vi "openLoopControlView.vi"(10 "UserEvents in":refnum<class "UserEvents.lvclass">) -> ()   [LabVIEW 2015, in "FAMTViews.lvlib"]
uses:
  FAMTViews.lvlib
  UserEvents/UserEvents.lvclass
  CommandFactory/CommandFactory.lvclass
  UserEvents/UserEvents.lvclass/UserEvents.ctl
  Typedefs/StateSelector.ctl
  Commands/StartOpenLoopScan/StartOpenLoopScan.lvclass
  Typedefs/CommandSelector.ctl
  Typedefs/FAMTTypedefs.lvlib
panel:
  in  "cancelOpenLoopScanIsTrue":bool
  in  "startOpenLoopScanIsTrue":bool
  in  "Center Point":dbl[unit]
  in  "Force Setpoint":dbl[unit]
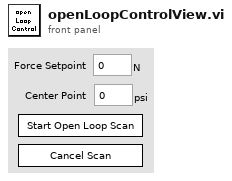
[diagram p1: front panel]
types:
  T1 = typedef "FAMTTypedefs.lvlib/PubDataEvents.ctl" = cluster{"State":refnum<user-event>, "ErrorCode":refnum<user-event>, "OutputData":refnum<user-event>, "InputData":refnum<user-event>, "ControllerData":refnum<user-event>, "TestStatus":refnum<user-event>, "LogPath":refnum<user-event>}
  T2 = typedef "FAMTTypedefs.lvlib/SubDataEvents.ctl" = cluster{"Command":refnum<user-event>}
  T3 = cluster{"Event Registration Refnum":refnum<event-registration>}
  T4 = typedef "FAMTTypedefs.lvlib/StateSelector.ctl" = enum16{"OfflineState", "FaultState", "StandbyState", "DisabledState", "EnabledState", "WaitForUserInputState", "PerformOpenLoopScanState"}
  T5 = typedef "FAMTTypedefs.lvlib/CommandSelector.ctl" = enum16{"Start", "Enable", "Disable", "Standby", "Shutdown"}
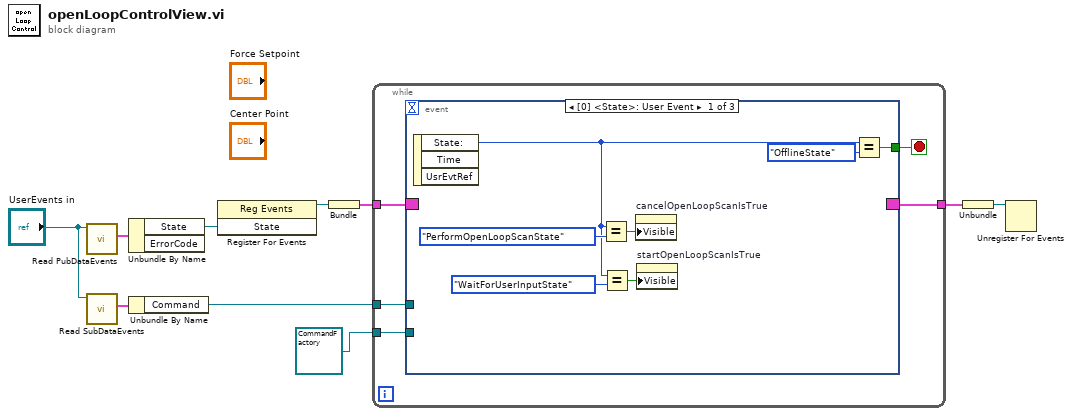
[diagram p0: block diagram]
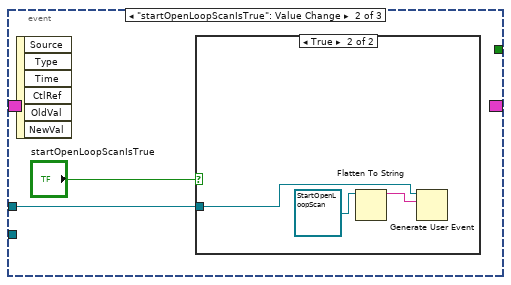
[diagram p2: hidden frame]
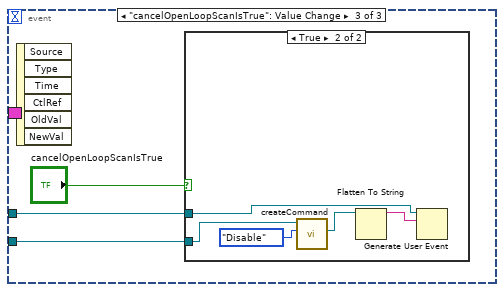
[diagram p4: hidden frame]
diagram:
  n1 = call "Read PubDataEvents.vi"("UserEvents in"="UserEvents in") -> ("PubDataEvents"=w10:T1)  [unwired: 9 in, 1 out]
  n2 = call "Read SubDataEvents.vi"("UserEvents in"="UserEvents in") -> ("SubDataEvents"=w4:T2)  [unwired: 9 in, 1 out]
  n3 = Unbundle By Name(w10) -> ("State"=w9:refnum<user-event>)  [unwired: 1 out]
  n4 = Unbundle By Name(w4) -> ("Command"=w2:refnum<user-event>)
  n5 = register-events(w9) -> (reference out=w8:refnum<event-registration>)  [unwired: 2 in, 1 out]
  n6 = Bundle("Event Registration Refnum"=w8) -> (w5:T3)  [unwired: 1 in]
  n7 = while {
    tunnel: w5 -> [w15]
    tunnel: [w14] -> w6
    tunnel: w2 -> [w12]
    tunnel: refnum<class "CommandFactory.lvclass"> refnum ("CommandFactory.lvclass") -> [w11]
    stop <- w13 stop-if-true
    n8 = event shown="[0] <State>: User Event" {
      selector: w15 -> [_ _ _]
      dyn-events: [_ _ _] -> w14
      timeout: _ -> [_ _ _]
      tunnel: [w21 _ _] -> w13
      tunnel: w12 -> [_ w23 w29]
      tunnel: w11 -> [_ _ w28]
      event User Event {
        n9 = event-data() -> ("State:"=w18:T4)  [unwired: 1 in, 2 out]
        n10 = Equal?(x=w18, y=StateSelector."PerformOpenLoopScanState") -> (x = y?=w17:bool)
        n11 = Equal?(x=w18, y=StateSelector."WaitForUserInputState") -> (x = y?=w16:bool)
        n12 = property on="cancelOpenLoopScanIsTrue" class="Bool"("Visible"=w17) -> ()  [unwired: 2 in, 2 out]
        n13 = property on="startOpenLoopScanIsTrue" class="Bool"("Visible"=w16) -> ()  [unwired: 2 in, 2 out]
        n14 = Equal?(x=w18, y=StateSelector."OfflineState") -> (x = y?=w21:bool)
      }
      event "startOpenLoopScanIsTrue": Value Change {
        n15 = event-data() -> ()  [unwired: 1 in, 6 out]
        n16 = case shown="True" "startOpenLoopScanIsTrue" {
          tunnel: w23 -> [_ w26]
          frame False {
          }
          frame True {
            n17 = Flatten To String(anything=refnum<class "StartOpenLoopScan.lvclass"> refnum ("StartOpenLoopScan.lvclass")) -> (data string=w27:string)  [unwired: 3 in, 2 out]
            n18 = Generate User Event(user event=w26, event data cluster=w27) -> ()  [unwired: 2 in, 2 out]
          }
        }
      }
      event "cancelOpenLoopScanIsTrue": Value Change {
        n19 = event-data() -> ()  [unwired: 1 in, 6 out]
        n20 = case shown="True" "cancelOpenLoopScanIsTrue" {
          tunnel: w29 -> [_ w34]
          tunnel: w28 -> [_ w31]
          frame False {
          }
          frame True {
            n21 = call-dynamic "createCommand.vi"("Command"=CommandSelector."Disable", "CommandFactory in"=w31) -> ("command"=w32:refnum<class "Command.lvclass">)  [unwired: 7 in, 2 out]
            n22 = Flatten To String(anything=w32) -> (data string=w35:string)  [unwired: 3 in, 2 out]
            n23 = Generate User Event(user event=w34, event data cluster=w35) -> ()  [unwired: 2 in, 2 out]
          }
        }
      }
    }
  }
  n24 = Unbundle(w6) -> ("Event Registration Refnum"=w7:refnum<event-registration>)
  n25 = Unregister For Events(event registration refnum=w7) -> ()  [unwired: 1 in, 1 out]
